vi "PatientSpecificFileNameGen2.vi"(2 "Location":T1, 3 "Add to Database":bool=TRUE, 4 "Done":bool, 5 "Auto Increment":bool=TRUE) -> (0 "SavePathOut":path, 1 "PatientFileName":string)   [LabVIEW 2022 SP3]
uses:
  LymphNodeInfo.ctl
  TissueTypeScan.ctl
  ScanningControl/-ScanSystem/Controls/location.ctl
  <vilib>/Utility/miscctls.llb/LVPositionTypeDef.ctl
  PatientGlobals.vi
panel:
  in  "Optional Suffix":string
  in  "Node Info":T2={"Patient Number"=0, "Node Set"="A", "Node Number"=0, "Tissue Type"=enum."Breast", "Tissue Location (Other)"="", "Node Classification"=enum."Whole Node", "Fresh?"=enum."Fresh?", "Year"=0} {"Year" format="%02d"; "Patient Number" format="%03d"; "Node Number" format="%02d"}
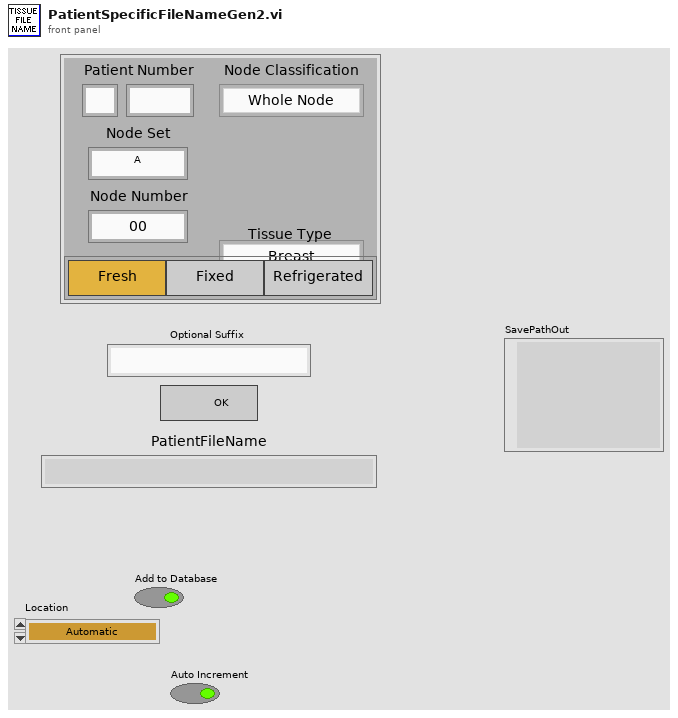
[diagram p1: front panel]
types:
  T1 = typedef "location.ctl" = enum16{"Automatic", "WCM Main", "Hawaii", "Columbia MM3000", "Columbia  NI System", "NYU", "RRI 2", "UHI Allen", "CUMC RT", "Chiba", "Stony Brook", "WCM Microscopy", "WCM Aeoretch", "WCM Optics Lab", "WCM Main 2Axis", "WCM Rotation", "WCM SAM SMAC", "SERI GP"}
  T2 = typedef "LymphNodeInfo.ctl" = cluster{"Patient Number":u32, "Node Set":string, "Node Number":u32, "Tissue Type":T3, "Tissue Location (Other)":string, "Node Classification":enum16{"Whole Node", "Piece A", "Piece B", "Piece C"}, "Fresh?":enum32{"Fresh?", "Fixed?", "Refrigerated?"}, "Year":u32}
  T3 = typedef "TissueTypeScan.ctl" = enum16{"Breast", "Gastric", "Stomach", "Rectal", "Colon", "Head & Neck", "Other"}
  T4 = typedef "LVPositionTypeDef.ctl" = cluster{"Left":i32, "Top":i32}
  T5 = typedef "ScannedNodeArray.ctl" = T2[]
  T6 = cluster{"Patient Number":bool, "Node Set":bool, "Node Number":bool, "Tissue Type":bool, "Tissue Location (Other)":bool, "Node Classification":bool, "Fresh?":bool, "Year":bool}
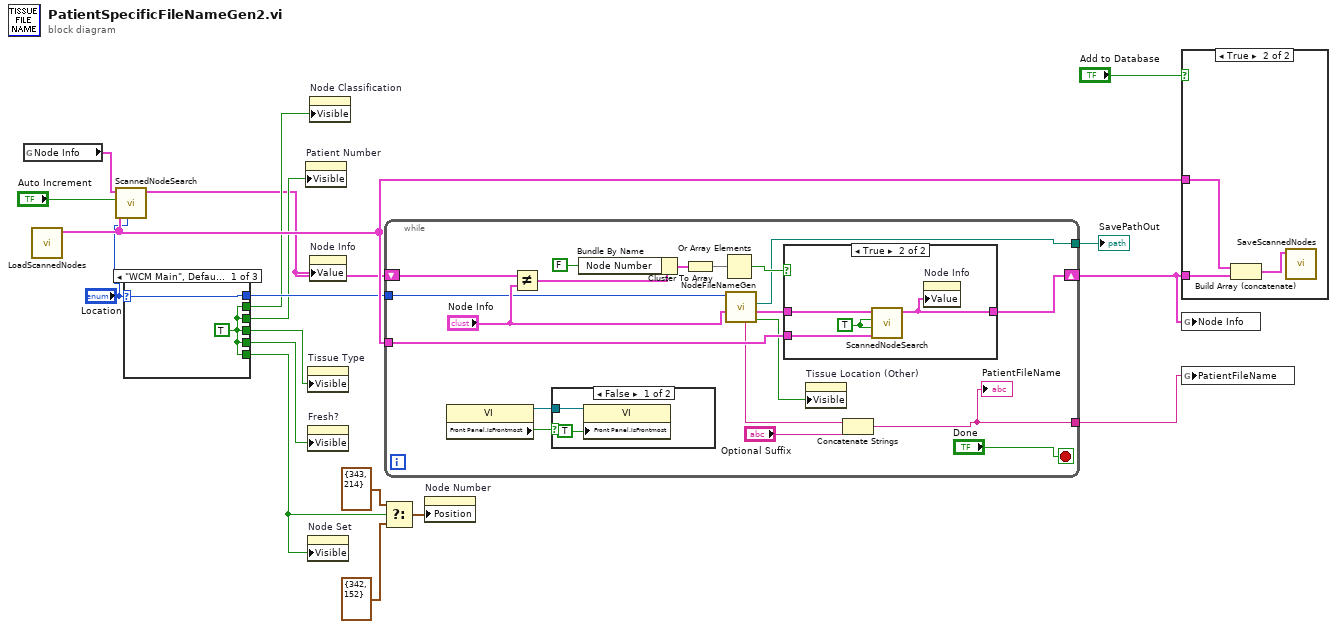
[diagram p0: block diagram]
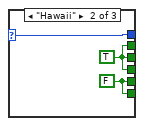
[diagram p2: hidden frame]
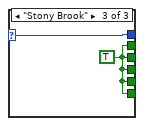
[diagram p3: hidden frame]
diagram:
  n1 = global read "PatientGlobals.vi" "Node Info"() -> (w18:T2)
  n2 = call "LoadScannedNodes.vi"() -> ("Previously Scanned Nodes"=w15:T5)  [unwired: 11 in]
  n3 = call "ScannedNodeSearch.vi"("Location"="Location", "Previously Scanned Nodes"=w15, "Auto Increment"="Auto Increment", "Searched Node"=w18) -> ("Next Node"=w2:T2)  [unwired: 7 in]
  n4 = case shown="\"WCM Main\", Default" "Location" {
    selector: "Location" -> [w20 w23 w25]
    tunnel: [w20 w23 w25] -> w12
    tunnel: [w19 w22 w24] -> w11
    tunnel: [w19 w22 w24] -> w10
    tunnel: [w19 w22 w24] -> w9
    tunnel: [w19 w21 w24] -> w7
    tunnel: [w19 w21 w24] -> w8
    frame "WCM Main", Default {
      w19 = TRUE
    }
    frame "Hawaii" {
      w21 = FALSE
      w22 = TRUE
    }
    frame "Stony Brook" {
      w24 = TRUE
    }
  }
  n5 = property on="Patient Number" class="DigNum (strict)"("Visible"=w11) -> ()  [unwired: 2 in, 2 out]
  n6 = property on="Tissue Type" class="Enum (strict)"("Visible"=w10) -> ()  [unwired: 2 in, 2 out]
  n7 = property on="Fresh?" class="RadioBtnsControl (strict)"("Visible"=w8) -> ()  [unwired: 2 in, 2 out]
  n8 = property on="Node Set" class="Str"("Visible"=w7) -> ()  [unwired: 2 in, 2 out]
  n9 = property on="Node Classification" class="Enum (strict)"("Visible"=w9) -> ()  [unwired: 2 in, 2 out]
  n10 = property on="Node Info" class="Clust (strict)"("Value"=w2) -> ()  [unwired: 2 in, 2 out]
  n11 = Select(t=T4 {"Left"=343, "Top"=214} ("Position"), s=w7, f=T4 {"Left"=342, "Top"=152} ("Position")) -> (s? t:f=w4:T4)
  n12 = while {
    tunnel: w15 -> [w43]
    shift-right: [w34] -> w13
    shift-left: w2 -> [w41]
    tunnel: [w26] -> w3
    tunnel: [w35] -> w14
    tunnel: w12 -> [w30]
    stop <- "Done" stop-if-true
    n13 = property class="VI"() -> (reference out=w29:refnum<vi>, "Front Panel.IsFrontmost"=w28:bool)  [unwired: 2 in, 1 out]
    n14 = Not Equal?(x=w41, y="Node Info") -> (x != y?=w42:T6)
    n15 = case shown="False" w28 {
      tunnel: w29 -> [w45 _]
      frame False {
        n16 = property class="VI"(reference=w45, "Front Panel.IsFrontmost"=TRUE) -> ()  [unwired: 1 in, 2 out]
      }
      frame True {
      }
    }
    n17 = Bundle By Name(cluster=w42, "Node Number"=FALSE) -> (w32:T6)
    n18 = Cluster To Array(cluster=w32) -> (array=w40:bool[])
    n19 = Or Array Elements(Boolean array=w40) -> (logical OR=w39:bool)
    n20 = call "NodeFileNameGen.vi"("Node Info in"="Node Info", "Location"=w30) -> ("Other Box Visible?"=w33:bool, "Node Info out"=w37:T2, "SavePathOut"=w35:path, "PatientFileName"=w36:string)  [unwired: 6 in]
    n21 = case shown="True" w39 {
      tunnel: w43 -> [_ w51]
      tunnel: w37 -> [w47 w50]
      tunnel: [w47 w48] -> w34
      frame False {
      }
      frame True {
        w49 = TRUE ("Auto Increment")
        n22 = call "ScannedNodeSearch.vi"("Previously Scanned Nodes"=w51, "Reset Node Count?"=w49, "Auto Increment"=w49, "Searched Node"=w50) -> ("Next Node"=w48:T2)  [unwired: 7 in]
        n23 = property on="Node Info" class="Clust (strict)"("Value"=w48) -> ()  [unwired: 2 in, 2 out]
      }
    }
    n24 = property on="Tissue Location (Other)" class="Str"("Visible"=w33) -> ()  [unwired: 2 in, 2 out]
    n25 = Concatenate Strings(w36, "Optional Suffix") -> (w26:string)
    "PatientFileName" <- w26
  }
  "SavePathOut" <- w14
  n26 = property on="Node Number" class="DigNum (strict)"("Position"=w4) -> ()  [unwired: 2 in, 2 out]
  n27 = case shown="True" "Add to Database" {
    tunnel: w13 -> [_ w54]
    tunnel: w15 -> [_ w52]
    frame False {
    }
    frame True {
      n28 = Build Array (concatenate)(w52, w54) -> (w53:T5)
      n29 = call "SaveScannedNodes.vi"("Scanned Nodes"=w53) -> ()  [unwired: 11 in]
    }
  }
  n30 = global write "PatientGlobals.vi" "Node Info"(w13) -> ()
  n31 = global write "PatientGlobals.vi" "PatientFileName"(w3) -> ()
